vi "Test_Machine_Etats.vi"() -> ()   [LabVIEW 2026]
doc: "Illustre les principes de base du modèle de conception de machine à états dans LabVIEW. Les machines à états les plus simples sont composées d'une structure Condition dans une boucle While, avec un énum d'états câblé à un registre à décalage de la boucle pour définir l'exécution des différentes conditions (ou \"états\") de la structure Condition à différentes itérations de la boucle."
uses:
  Etats.ctl
panel:
  out "error out":errorcluster caption="sortie d'erreur"
  in  "error in":errorcluster caption="entrée d'erreur"
  in  "Arrêter":bool
  in  "Exécuter l'état 2":bool
  in  "Exécuter l'état 1":bool
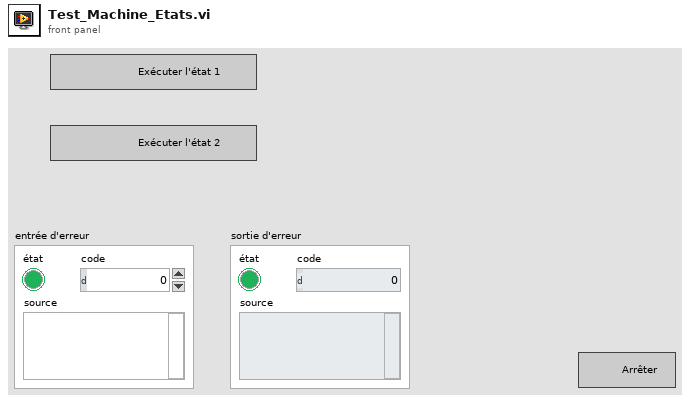
[diagram p1: front panel]
types:
  T1 = typedef "Etats.ctl" = enum16{"Initialize", "TEST", "Wait for Event", "Convert", "Move", "State 2", "State 3", "Stop"}
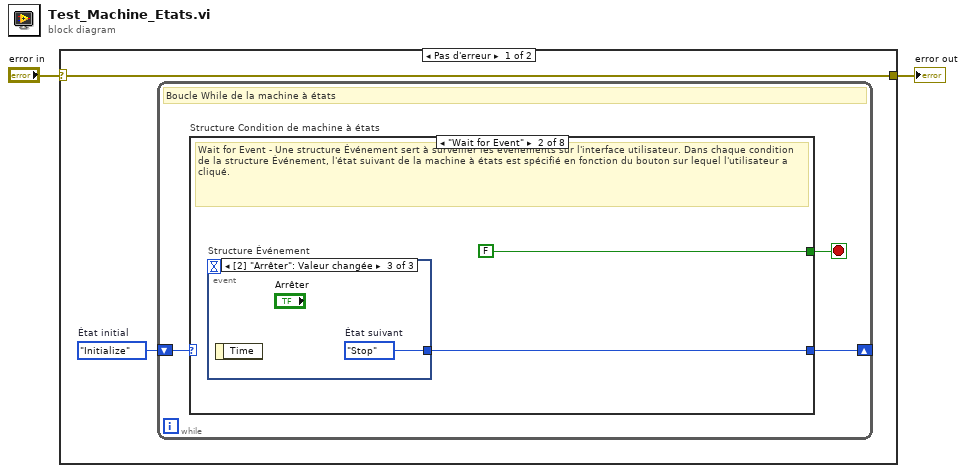
[diagram p0: block diagram]
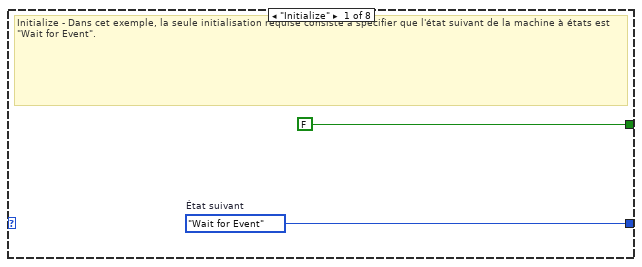
[diagram p2: hidden frame]
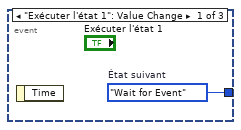
[diagram p3: hidden frame]
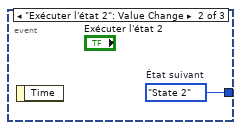
[diagram p4: hidden frame]
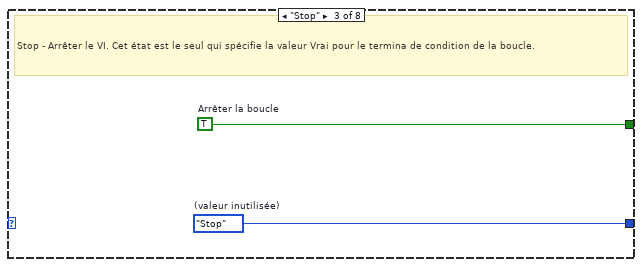
[diagram p5: hidden frame]
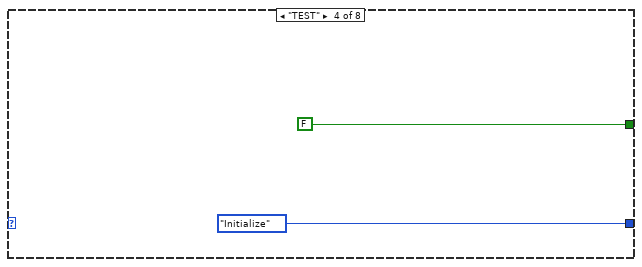
[diagram p6: hidden frame]
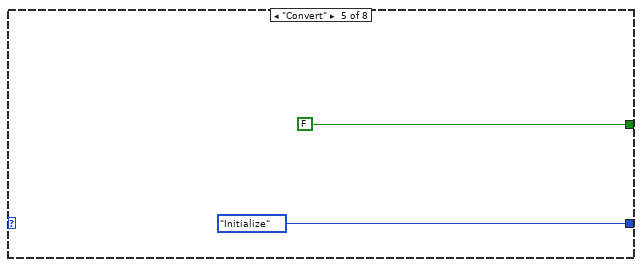
[diagram p7: hidden frame]
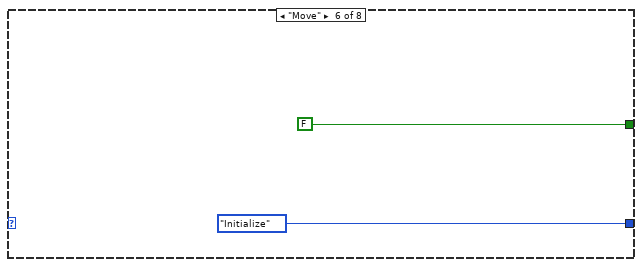
[diagram p8: hidden frame]
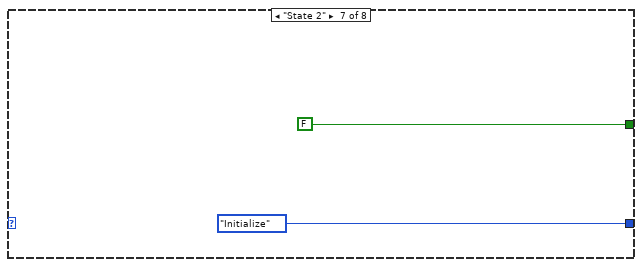
[diagram p9: hidden frame]
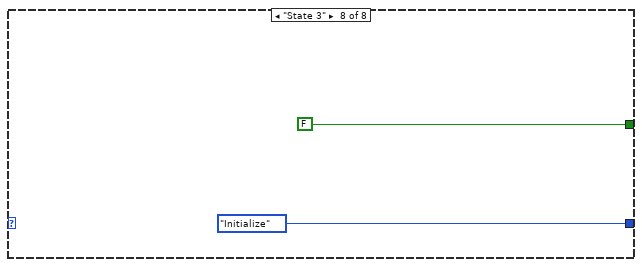
[diagram p10: hidden frame]
diagram:
  n1 = case shown="Pas d'erreur" "error in" {
    selector: "error in" -> [w3 w27]
    tunnel: [w3 w27] -> w1
    frame No Error {
      w4 = Etats."Initialize"  # État initial
      n2 = while {
        shift-right: [w6] -> _
        shift-left: w4 -> [w7]
        stop <- w5 stop-if-true
        # "Boucle While de la machine à états"
        n3 = case "Structure Condition de machine à états" shown="\"Wait for Event\"" w7 {
          tunnel: [w9 w11 w16 Etats."Initialize" ("(valeur inutilisée)") Etats."Initialize" ("(valeur inutilisée)") Etats."Initialize" ("(valeur inutilisée)") Etats."Initialize" ("(valeur inutilisée)") Etats."Initialize" ("(valeur inutilisée)")] -> w6
          tunnel: [FALSE ("Arrêter la boucle") FALSE ("Arrêter la boucle") w15 FALSE ("Arrêter la boucle") FALSE ("Arrêter la boucle") FALSE ("Arrêter la boucle") FALSE ("Arrêter la boucle") FALSE ("Arrêter la boucle")] -> w5
          frame "Initialize" {
            w9 = Etats."Wait for Event"  # État suivant
            # "Initialize - Dans cet exemple, la seule initialisation requise consiste à spécifier que l'état suivant de la machine à états est \"Wait for Event\"."
          }
          frame "Wait for Event" {
            # "Wait for Event - Une structure Événement sert à surveiller les événements sur l'interface utilisateur. Dans chaque condition de la structure Événement, l'état suivant de la machine à états est spécifié en fonction du bouton sur lequel l'utilisateur a cliqué."
            n4 = event "Structure Événement" shown="[2] \"Arrêter\": Valeur changée" {
              selector: _ -> [_ _ _]
              dyn-events: _ -> [_ _ _]
              timeout: _ -> [_ _ _]
              tunnel: [w12 w13 w14] -> w11
              event "Exécuter l'état 1": Value Change {
                w12 = Etats."Wait for Event"  # État suivant
                n5 = event-data() -> ()  [unwired: 1 in, 1 out]
              }
              event "Exécuter l'état 2": Value Change {
                w13 = Etats."State 2"  # État suivant
                n6 = event-data() -> ()  [unwired: 1 in, 1 out]
              }
              event "Arrêter": Value Change {
                w14 = Etats."Stop"  # État suivant
                n7 = event-data() -> ()  [unwired: 1 in, 1 out]
              }
            }
          }
          frame "Stop" {
            w15 = TRUE  # Arrêter la boucle
            w16 = Etats."Stop"  # (valeur inutilisée)
            # "Stop - Arrêter le VI. Cet état est le seul qui spécifie la valeur Vrai pour le termina de condition de la boucle."
          }
          frame "TEST" {
          }
          frame "Convert" {
          }
          frame "Move" {
          }
          frame "State 2" {
          }
          frame "State 3" {
          }
        }
      }
    }
    frame Error {
    }
  }
  "error out" <- w1
